vi "Read Descr.vi"(8 "error in (no error)":errorcluster, 11 "CRDS Cell in":refnum<class "CRDS Cell.lvclass">) -> (0 "error out":errorcluster, 2 "Descr":T1, 3 "CRDS Cell out":refnum<class "CRDS Cell.lvclass">)   [LabVIEW 2011]
doc: "Retrieve the description of the cell. The cell can be a reference (i.e. gas phase only), dry or humidified)."
uses:
  CRDS Cell.lvclass
  PAS_CRDS new/CRDS/Controls/chDescr.ctl
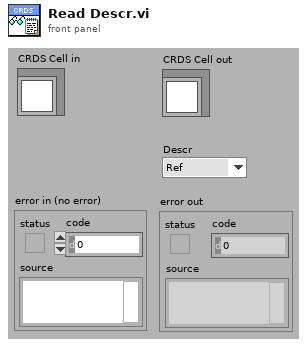
[diagram p1: front panel]
types:
  T1 = typedef "chDescr.ctl" = enum16{"Ref", "Dry", "60%", "90%"}
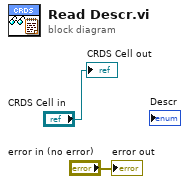
[diagram p0: block diagram]
diagram:
  "error out" <- "error in (no error)"
  "CRDS Cell out" <- "CRDS Cell in"
